vi "tmp 2D float to bytes.vi"(6 "kwarg_name":string, 8 "error in (no error)":errorcluster, 10 "Bindata & descr in":T1, 11 "data in":dbl[][](array[numeric])) -> (0 "error out":errorcluster, 2 "Bindata & descr out":T1, 3 "flattened data out":dbl[](array[numeric]))   [LabVIEW 2018]
uses:
  Bindata&description.ctl
  Bindata description.ctl
  8fae7cd3-ef5a-444d-abab-9196454fa199.vi
  8fae7cd3-ef5a-444d-abab-9196454fa199.vi/3feffd84-2a14-46ec-a4a3-85f8de9c3cde.vi
  8fae7cd3-ef5a-444d-abab-9196454fa199.vi/3feffd84-2a14-46ec-a4a3-85f8de9c3cde.vi/d0fee912-6c67-4b55-bc0a-a65a21ef5c35.vi
  LV-Julia_ZMQ-Roundtrip_lib.lvlib
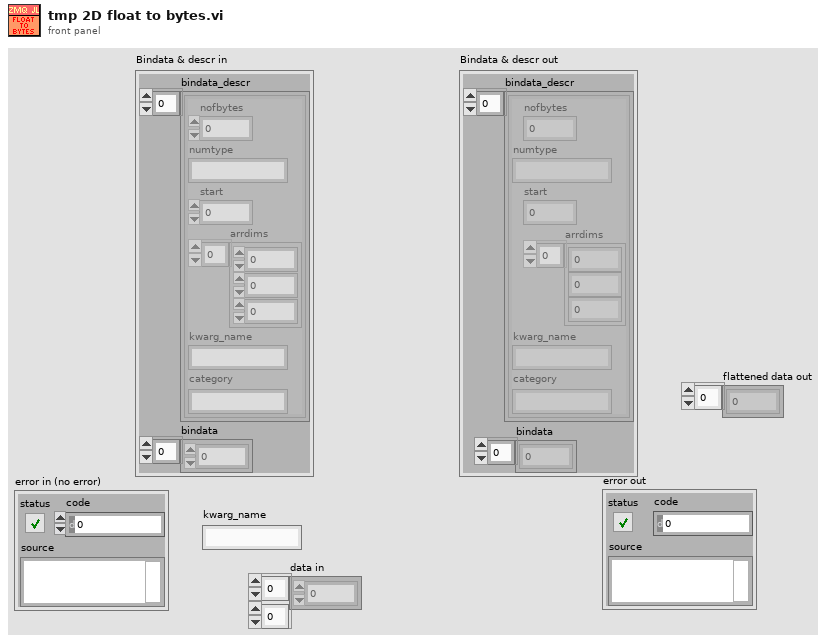
[diagram p1: front panel]
types:
  T1 = typedef "Bindata&description.ctl" = cluster{"bindata_descr":T2[], "bindata":u8[]}
  T2 = typedef "LV-Julia_ZMQ-Roundtrip_lib.lvlib/Bindata description.ctl" = cluster{"nofbytes":i32, "numtype":string, "start":i32, "arrdims":i32[], "kwarg_name":string, "category":string}
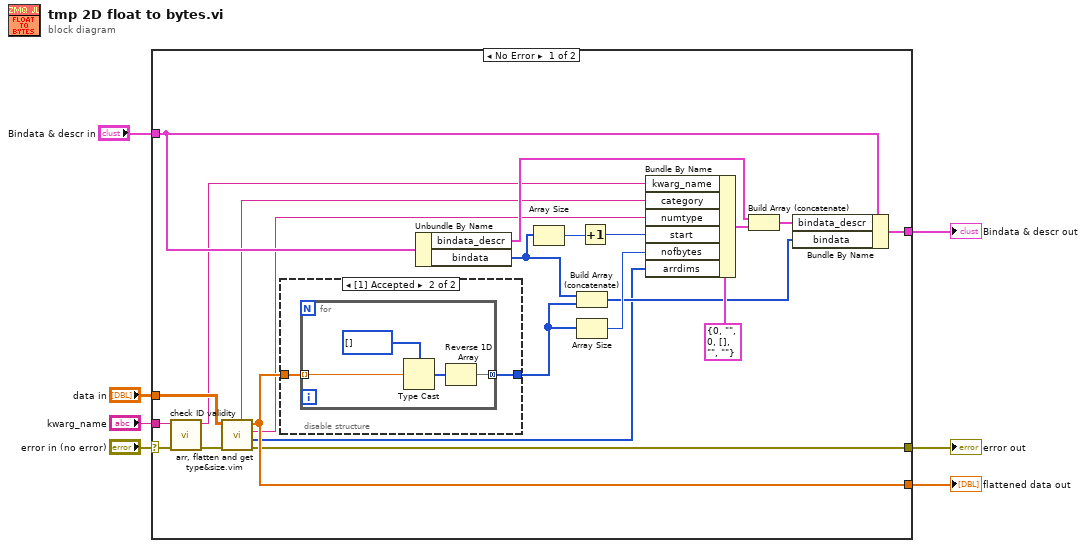
[diagram p0: block diagram]
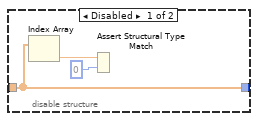
[diagram p2: hidden frame]
diagram:
  n1 = case shown="No Error" "error in (no error)" {
    selector: "error in (no error)" -> [w22 w39]
    tunnel: "data in" -> [w24 _]
    tunnel: [w23 _] -> w6
    tunnel: "kwarg_name" -> [w21 _]
    tunnel: "Bindata & descr in" -> [w20 _]
    tunnel: [w18 _] -> w2
    tunnel: [w13 w39] -> w1
    frame No Error {
      n2 = call "check ID validity.vi"("error in (no error)"=w22, "ID in"=w21) -> ("error out"=w12:errorcluster, "ID out"=w9:string)  [unwired: 8 in]
      n3 = call "arr, flatten and get type&size.vim"("error in (no error)"=w12, "data in"=w24) -> ("error out"=w13:errorcluster, "sizes"=w11:i32[], "numtype"=w10:string, "flattened array out"=w23:dbl[], "category"=w8:string)  [unwired: 5 in]
      n4 = disable-structure shown="[1] Accepted" {
        disable-tunnel: [w30 w34] -> w29
        disable-tunnel: w23 -> [w30 w33]
        frame Disabled {
          n5 = Index Array(array=w30) -> (element=w32:dbl)  [unwired: 1 in]
          n6 = Assert Structural Type Match(0:u8 0 ("element"), 1:w32) -> ()
        }
        frame Enabled {
          n7 = for {
            tunnel: w33 -> [w37] mode=indexing
            tunnel: [w38] -> w34 mode=concatenating
            n8 = Type Cast(type=u8[] [], x=w37) -> (*(type *) &x=w35:u8[])
            n9 = Reverse 1D Array(array=w35) -> (reversed array=w38:u8[])
          }
        }
      }
      n10 = Unbundle By Name(w20) -> ("bindata_descr"=w16:T2[], "bindata"=w19:u8[])
      n11 = Array Size(array=w19) -> (size(s)=w28:i32)
      n12 = Build Array (concatenate)(w19, w29) -> (w17:u8[])
      n13 = Array Size(array=w29) -> (size(s)=w25:i32)
      n14 = Increment(x=w28) -> (x+1=w26:i32)
      n15 = Bundle By Name(cluster=T2 {"nofbytes"=0, "numtype"="", "start"=0, "arrdims"=[], "kwarg_name"="", "category"=""} ("bindata descr"), "kwarg_name"=w9, "category"=w8, "numtype"=w10, "start"=w26, "nofbytes"=w25, "arrdims"=w11) -> (w14:T2)
      n16 = Build Array (concatenate)(w16, w14) -> (w15:T2[])
      n17 = Bundle By Name(cluster=w20, "bindata_descr"=w15, "bindata"=w17) -> (w18:T1)
    }
    frame Error {
    }
  }
  "flattened data out" <- w6
  "error out" <- w1
  "Bindata & descr out" <- w2
